vi "Inject Attribute List.vi"(6 "Attributes Ref":refnum<data-value>, 8 "error in (no error)":errorcluster, 11 "Start Bug Remover in":refnum<class "Start Bug Remover.lvclass">) -> (0 "error out":errorcluster, 3 "Start Bug Remover out":refnum<class "Start Bug Remover.lvclass">)   [LabVIEW 2019, in "Start Bug Remover.lvclass"]
uses:
  <vilib>/gpm_packages/@cs/Car-wash/Source/Process Steps/Start Bug Remover/Start Bug Remover.lvclass
  <vilib>/gpm_packages/@cs/lookup-table/Source/LookupTable/LookupTable.lvclass
  <vilib>/gpm_packages/@cs/lookup-table/Source/LookupTable/LookupTable.lvclass/LookupTable.ctl
  <vilib>/gpm_packages/@cs/Car-wash/Source/Process Steps/Start Bug Remover/Start Bug Remover.lvclass/Start Bug Remover.ctl
  15c55689-809c-4f32-84df-62098553d5d4.vi
  <vilib>/gpm_packages/@cs/lookup-table/Source/LookupTable/Read Table Reference.vi
  15c55689-809c-4f32-84df-62098553d5d4.vi/77fb5852-0cdc-4744-8573-97092178236c.vi
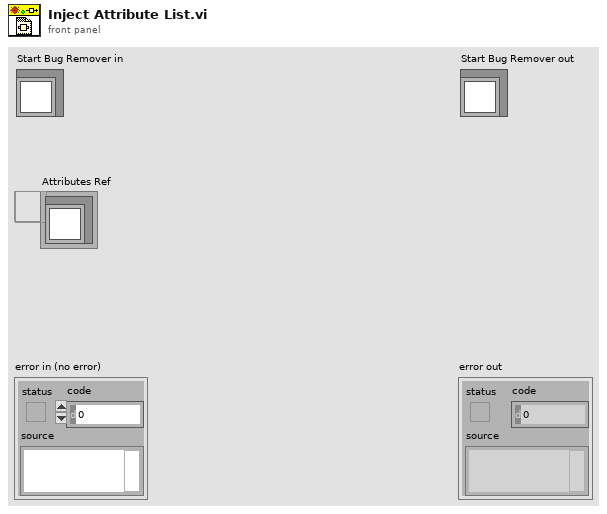
[diagram p1: front panel]
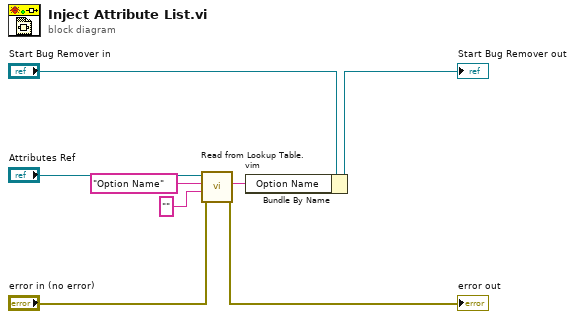
[diagram p0: block diagram]
diagram:
  n1 = call "Read from Lookup Table.vim"("error in (no error)"="error in (no error)", "Type"="", "Item Name"="Option Name", "LookupTable Reference"="Attributes Ref") -> ("error out"=→"error out":errorcluster, "Value"=w6:string)  [unwired: 4 in, 2 out]
  n2 = Bundle By Name(cluster="Start Bug Remover in", "Option Name"=w6) -> (→"Start Bug Remover out":refnum<class "Start Bug Remover.lvclass">)
